vi "Write Outputs to System.vi"(8 "error in (no error)":errorcluster, 10 "Data In":dbl[](array[numeric]), 11 "Channel Data References":T1[](array[typedef]) format="%.0x") -> (0 "error out":errorcluster, 2 "Data Out":dbl[](array[numeric]))   [LabVIEW 2021]
uses:
  <vilib>/NI VeriStand/Custom Device API/Data Reference.ctl
  <vilib>/NI VeriStand/Custom Device API/Global Data Refs.vi
  <vilib>/NI VeriStand/Custom Device API/Custom Device API.lvlib
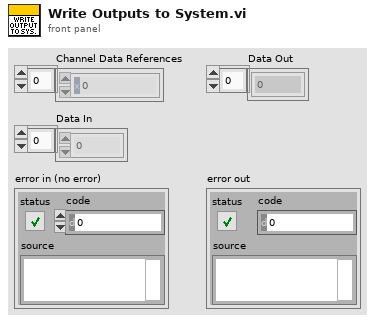
[diagram p1: front panel]
types:
  T1 = typedef "Custom Device API.lvlib/Data Reference.ctl" = i32
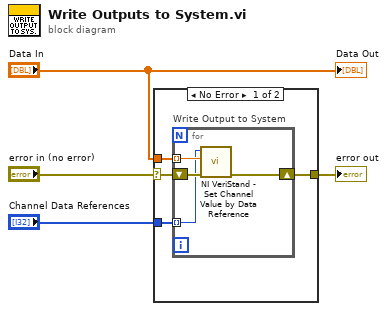
[diagram p0: block diagram]
diagram:
  n1 = case shown="No Error" "error in (no error)" {
    selector: "error in (no error)" -> [w8 w13]
    tunnel: "Data In" -> [w7 _]
    tunnel: [w6 w13] -> w2
    tunnel: "Channel Data References" -> [w5 _]
    frame No Error {
      n2 = for "Write Output to System" {
        shift-right: [w11] -> w6
        shift-left: w8 -> [w12]
        tunnel: w7 -> [w10] mode=indexing
        tunnel: w5 -> [w9] mode=indexing
        n3 = call <vilib>:"NI VeriStand - Set Channel Value by Data Reference.vi"("error in (no error)"=w12, "Value"=w10, "Data Reference in"=w9) -> ("error out"=w11:errorcluster)  [unwired: 8 out]
      }
    }
    frame Error {
    }
  }
  "error out" <- w2
  "Data Out" <- "Data In"
